vi "RT_Reboot.vi"() -> ()   [LabVIEW 2018]
uses:
  RT/PublicSubVI/Ctl/_ctl_RT_Working_State.ctl
  <vilib>/Utility/miscctls.llb/LVComboBoxStrsAndValuesArrayTypeDef.ctl
panel:
  in  "Cancel":bool
  in  "Reboot":bool
  in  "Select Reboot State":string(combo)="Working"
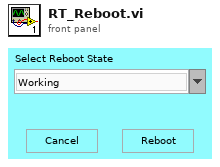
[diagram p1: front panel]
types:
  T1 = typedef "LVComboBoxStrsAndValuesArrayTypeDef.ctl" = cluster{"String":string, "Value":string}[]
  T2 = typedef "_ctl_RT_Working_State.ctl" = enum16{"Initialize", "Running", "Reboot_Work", "Reboot_Safe"}
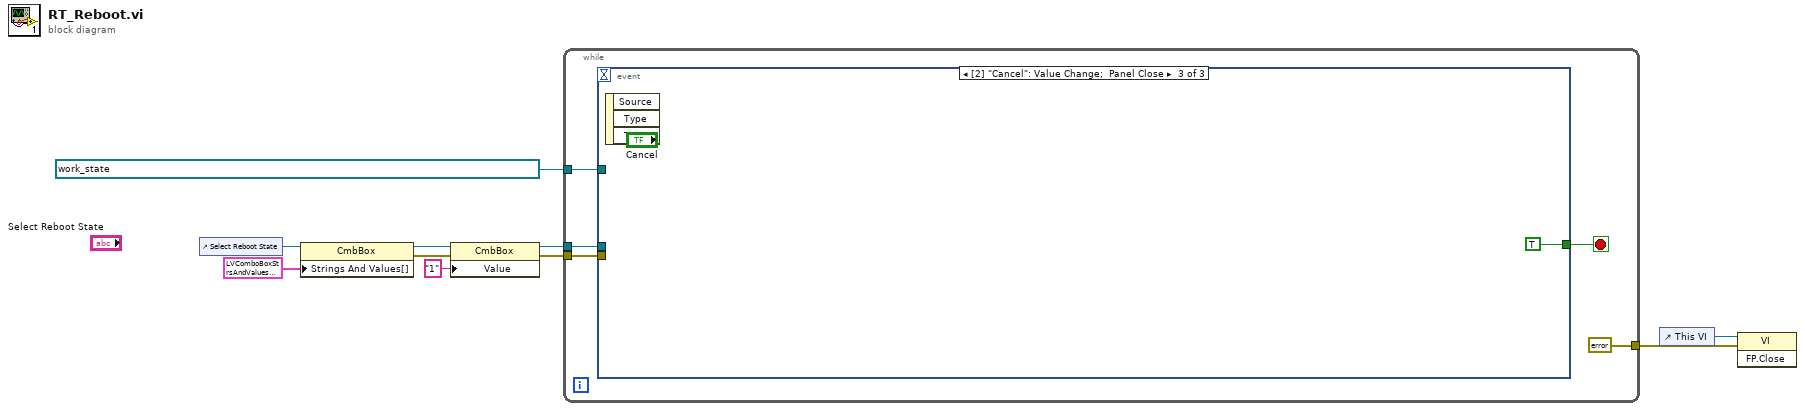
[diagram p0: block diagram]
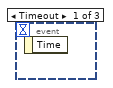
[diagram p2: hidden frame]
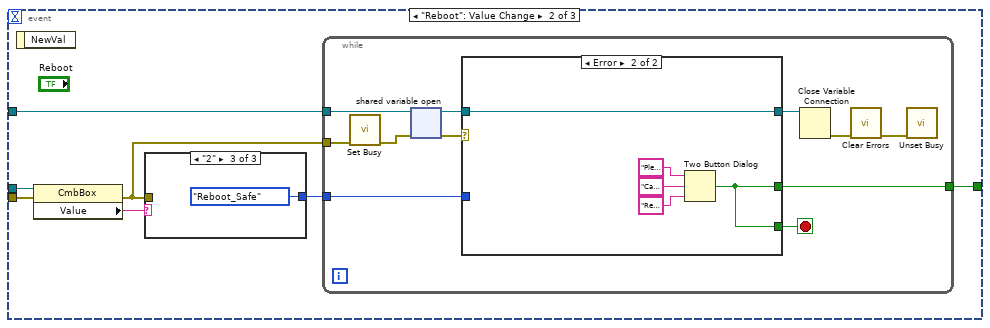
[diagram p3: hidden frame]
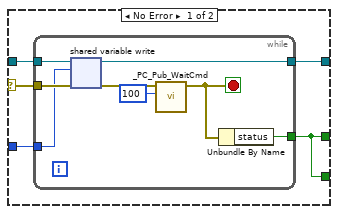
[diagram p4: hidden frame]
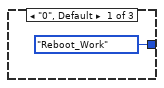
[diagram p5: hidden frame]
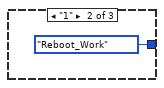
[diagram p6: hidden frame]
diagram:
  w3 = refnum<k21> "ni.var.psp://NI-sbRIO/_RT_CtrlLoop_Reboot_Monitor_Variable/RT_Working_State" items=["Initialize", "Running", "Reboot_Work", "Reboot_Safe"] ("shared variable refnum in")
  n1 = control-ref of="Select Reboot State"() -> (w10:refnum<vi>)
  n2 = property class="CmbBox"(reference=w10, "Strings And Values[]"=T1 [{"String"="Working", "Value"="1"}, {"String"="Safe", "Value"="2"}] ("Strings And Values []")) -> (reference out=w8:refnum<vi>, error out=w7:errorcluster)  [unwired: 1 in]
  n3 = property class="CmbBox"(reference=w8, error in=w7, "Value"="1") -> (reference out=w6:refnum<vi>, error out=w5:errorcluster)
  n4 = while {
    tunnel: w6 -> [w14]
    tunnel: w5 -> [w13]
    tunnel: w3 -> [w12]
    tunnel: [errorcluster {"status"=FALSE, "code"=0, "source"=""} ("error constant")] -> w1
    stop <- w15 stop-if-true
    n5 = event shown="[2] \"Cancel\": Value Change;  Panel Close" {
      selector: _ -> [_ _ _]
      dyn-events: _ -> [_ _ _]
      timeout: _ -> [_ _ _]
      tunnel: [_ w16 TRUE ("true")] -> w15
      tunnel: w14 -> [_ w22 _]
      tunnel: w13 -> [_ w21 _]
      tunnel: w12 -> [_ w18 _]
      event Timeout {
        n6 = event-data() -> ()  [unwired: 1 in, 1 out]
      }
      event "Reboot": Value Change {
        n7 = event-data() -> ()  [unwired: 1 in, 1 out]
        n8 = property class="CmbBox"(reference=w22, error in=w21) -> (error out=w17:errorcluster, "Value"=w20:string)  [unwired: 1 out]
        n9 = case shown="\"2\"" w20 {
          tunnel: w17 -> [_ _ _]
          tunnel: [_ctl_RT_Working_State."Reboot_Work" ("data in") _ctl_RT_Working_State."Reboot_Work" ("data in") _ctl_RT_Working_State."Reboot_Safe" ("data in")] -> w19
          frame "0", Default {
          }
          frame "1" {
          }
          frame "2" {
          }
        }
        n10 = while {
          tunnel: w19 -> [w33]
          tunnel: w18 -> [w30]
          tunnel: w17 -> [w25]
          tunnel: [w23] -> w16
          stop <- w24 stop-if-true
          n11 = call <vilib>:"Set Busy.vi"("error in (no error)"=w25) -> ("error out"=w29:errorcluster)  [unwired: 9 in, 1 out]
          n12 = shared-variable-open(w30, w29) -> (w32:refnum<k21>, w28:errorcluster)
          n13 = case shown="Error" w28 {
            selector: w28 -> [w35 _]
            tunnel: w33 -> [w38 _]
            tunnel: w32 -> [w37 w51]
            tunnel: [w36 w51] -> w31
            tunnel: [w34 w47] -> w24
            tunnel: [w34 w47] -> w23
            frame No Error {
              n14 = while {
                tunnel: w35 -> [w46]
                tunnel: w38 -> [w43]
                tunnel: w37 -> [w42]
                tunnel: [w41] -> w36
                tunnel: [w39] -> w34
                stop <- w40 stop-if-true
                n15 = shared-variable-write(w42, w46, w43) -> (w41:refnum<k21>, w44:errorcluster)
                n16 = call "_PC_Pub_WaitCmd.vi"("milliseconds to wait"=u32 100, "error in (no error)"=w44) -> ("error out"=w40:errorcluster)  [unwired: 9 in]
                n17 = Unbundle By Name(w40) -> ("status"=w39:bool)
              }
            }
            frame Error {
              n18 = Two Button Dialog(message="Please confirm the system connection status", 1:"ReConfirm Reboot" ("F button name (\"Cancel\")"), 2:"Cancel Reboot" ("T button name (\"OK\")")) -> (T button?=w47:bool)
            }
          }
          n19 = Close Variable Connection(11:w31) -> (0:w27:errorcluster)  [unwired: 1 in]
          n20 = call <vilib>:"Clear Errors.vi"("error in (no error)"=w27) -> ("error out"=w26:errorcluster)  [unwired: 5 in, 1 out]
          n21 = call <vilib>:"Unset Busy.vi"("error in (no error)"=w26) -> ()  [unwired: 10 in, 1 out]
        }
      }
      event "Cancel": Value Change; Panel Close {
        n22 = event-data() -> ()  [unwired: 1 in, 3 out]
      }
    }
  }
  n23 = control-ref of="This VI"() -> (w2:refnum<vi>)
  n24 = invoke class="VI" method="FP.Close"(reference=w2, error in=w1) -> ()  [unwired: 1 in, 3 out]
